vi "Generate_Start_or_Goal_District_Array .vi"(9 "District Name Array":string[](array[string]), 11 "Start_Goal District":string) -> (2 "Compare District Array":dbl[](array[numeric]))   [LabVIEW 2014]
doc: "产生起点到终点的节点数组"
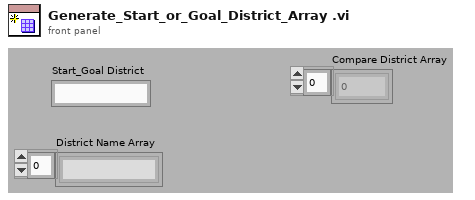
[diagram p1: front panel]
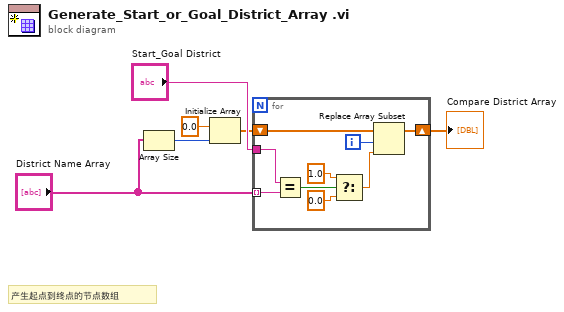
[diagram p0: block diagram]
diagram:
  # "产生起点到终点的节点数组"
  n1 = Array Size(array="District Name Array") -> (size(s)=w6:i32)
  n2 = Initialize Array(0.0 ("元素"), w6) -> (w2:dbl[])
  n3 = for {
    tunnel: "District Name Array" -> [w14] mode=indexing
    tunnel: "Start_Goal District" -> [w15]
    shift-right: [w9] -> w1
    shift-left: w2 -> [w10]
    i -> [w8]
    n4 = Equal?(x=w15, y=w14) -> (x = y?=w13:bool)
    n5 = Select(t=1.0, s=w13, f=0.0) -> (s? t:f=w7:dbl)
    n6 = Replace Array Subset(array=w10, new element=w7, index=w8) -> (w9:dbl[])
  }
  "Compare District Array" <- w1
